vi "Add Parameter.vi"(8 "error in":errorcluster, 10 "parameter configuration":T1 {"encoding" items=["BNR", "BCD", "Discrete"]}, 11 "message in":refnum<k24>) -> (0 "error out":errorcluster, 2 "new parameter":refnum<k24>, 3 "message out":refnum<k24>)   [LabVIEW 2020, in "AIM_1553_Parameter_ni.lvlib"]
uses:
  AIM_1553_Parameter_ni.lvlib
  C:/Users/Administrator/Desktop/GIT/Ballard-Arinc-429-XML-Generator/Source/Assemblies/Aim_1553_Parameter_ni/bin/Debug/AIM_1553_Parameter_ni.dll
  Assemblies/Aim_1553_Parameter_ni/bin/Debug/AIM_1553_Parameter_ni.dll
  _tyedefs/parameter_type.ctl
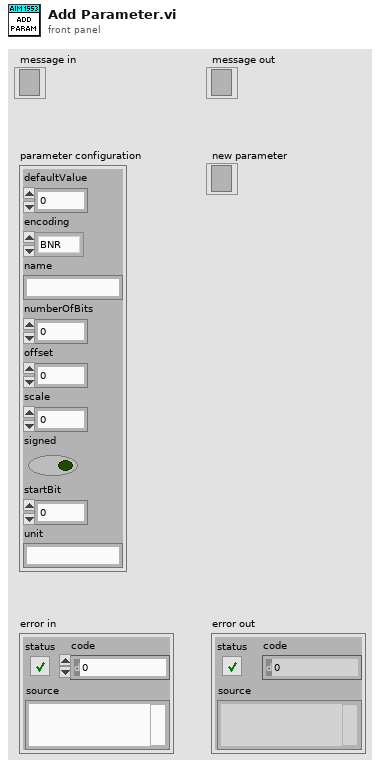
[diagram p1: front panel]
types:
  T1 = typedef "AIM_1553_Parameter_ni.lvlib/parameter_type.ctl" = cluster{"defaultValue":dbl, "encoding":i32, "name":string, "numberOfBits":i32, "offset":dbl, "scale":dbl, "signed":bool, "startBit":i32, "unit":string}
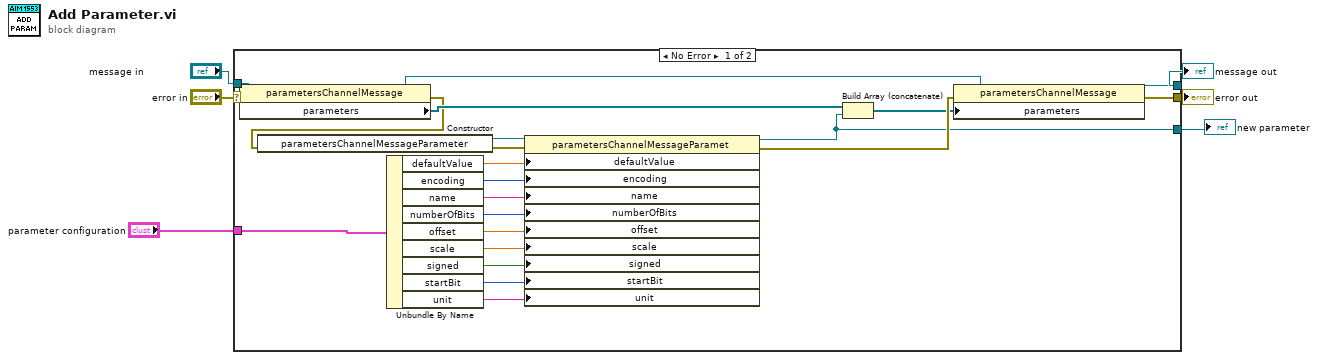
[diagram p0: block diagram]
diagram:
  n1 = case shown="No Error" "error in" {
    selector: "error in" -> [w27 w29]
    tunnel: [w25 w30] -> w6
    tunnel: [w24 w29] -> w5
    tunnel: "message in" -> [w28 w30]
    tunnel: "parameter configuration" -> [w17 _]
    tunnel: [w7 _] -> w1
    frame No Error {
      n2 = property class="parametersChannelMessage"(reference=w28, error in=w27) -> (reference out=w26:refnum<k24>, error out=w21:errorcluster, "parameters"=w22:refnum<k24>[])
      n3 = constructor class="parametersChannelMessageParamet"(error in=w21) -> (reference out=w23:refnum<k24>, error out=w20:errorcluster)  [unwired: 2 in, 1 out]
      n4 = Unbundle By Name(w17) -> ("defaultValue"=w16:dbl, "encoding"=w15:i32, "name"=w14:string, "numberOfBits"=w13:i32, "offset"=w12:dbl, "scale"=w11:dbl, "signed"=w10:bool, "startBit"=w9:i32, "unit"=w8:string)
      n5 = property class="parametersChannelMessageParamet"(reference=w23, error in=w20, "defaultValue"=w16, "encoding"=w15, "name"=w14, "numberOfBits"=w13, "offset"=w12, "scale"=w11, "signed"=w10, "startBit"=w9, "unit"=w8) -> (reference out=w7:refnum<k24>, error out=w19:errorcluster)
      n6 = Build Array (concatenate)(w22, w7) -> (w18:refnum<k24>[])
      n7 = property class="parametersChannelMessage"(reference=w26, error in=w19, "parameters"=w18) -> (reference out=w25:refnum<k24>, error out=w24:errorcluster)
    }
    frame Error {
    }
  }
  "message out" <- w6
  "error out" <- w5
  "new parameter" <- w1
